vi "CreatePaddle.vi"(8 "error in (no error)":errorcluster, 11 "class data in":refnum<class "Paddle.lvclass">) -> (0 "error out":errorcluster, 3 "class data out":refnum<class "Paddle.lvclass">)   [LabVIEW 2010, in "Labricks.lvlib" / "Paddle.lvclass"]
uses:
  Paddle.lvclass
  <vilib>/picture/3D Picture Control/NI_3D Picture Control.lvlib
  RenderBase/SceneObject_class/SceneObject.lvclass
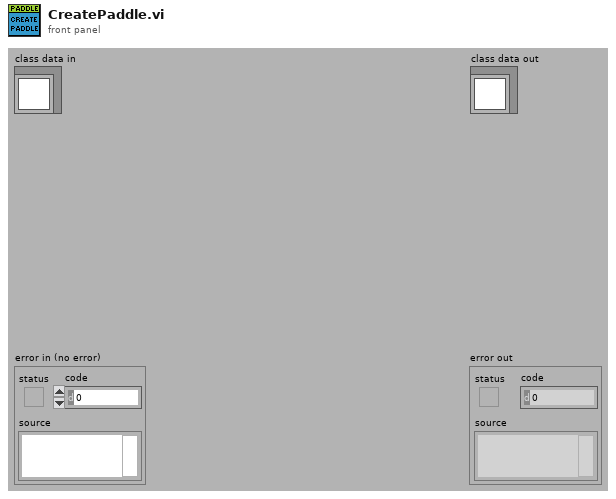
[diagram p1: front panel]
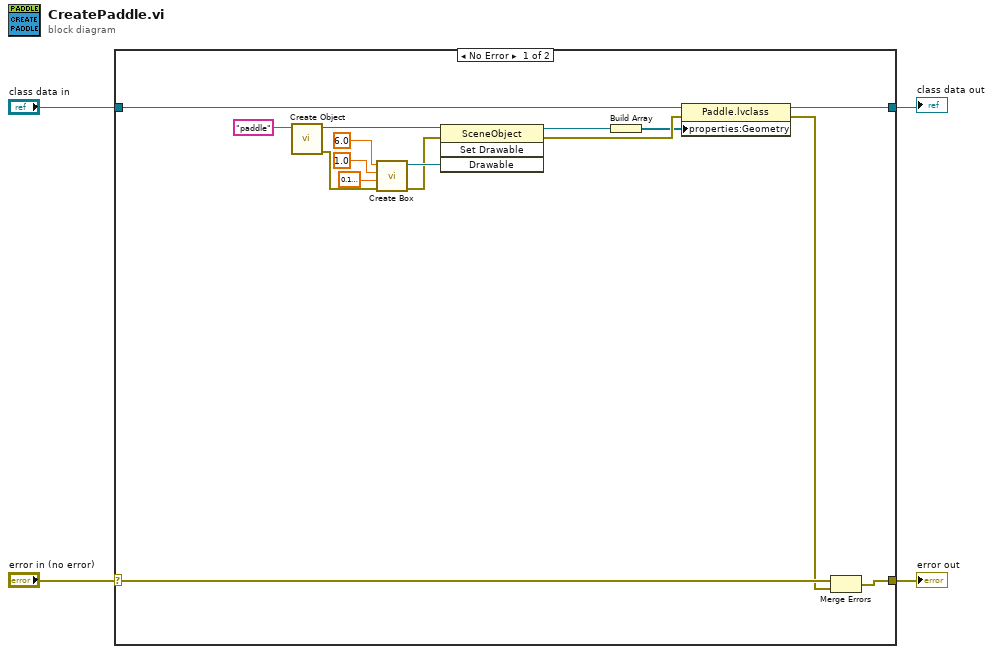
[diagram p0: block diagram]
diagram:
  n1 = case shown="No Error" "error in (no error)" {
    selector: "error in (no error)" -> [w20 w22]
    tunnel: [w17 w22] -> w3
    tunnel: "class data in" -> [w19 w21]
    tunnel: [w18 w21] -> w1
    frame No Error {
      n2 = call <vilib>:"Create Object.vi"("Name"="paddle") -> ("error out"=w10:errorcluster, "Scene:New Object"=w11:refnum<vi>)  [unwired: 9 in]
      n3 = call <vilib>:"Create Box.vi"("error in (no error)"=w10, "Length Z"=sgl 0.1, "Length Y"=sgl 1.0, "Length X"=sgl 6.0) -> ("error out"=w9:errorcluster, "New Box Refnum"=w12:refnum<vi>)  [unwired: 6 in]
      n4 = invoke class="SceneObject" method="Set Drawable"(reference=w11, error in=w9, "Drawable"=w12) -> (reference out=w6:refnum<vi>, error out=w7:errorcluster)  [unwired: 1 in, 2 out]
      n5 = Build Array(w6) -> (w5:refnum<vi>[])
      n6 = property class="Paddle.lvclass"(reference=w19, error in=w7, "properties:Geometry"=w5) -> (reference out=w18:refnum<class "Paddle.lvclass">, error out=w16:errorcluster)
      n7 = Merge Errors(w20, w16) -> (w17:errorcluster)
    }
    frame Error {
    }
  }
  "error out" <- w3
  "class data out" <- w1
